vi "getData.vi"(10 "TVAC Labview":bool, 11 "Local Debug":bool) -> ()   [LabVIEW 2017]
uses:
  <vilib>/httpClient/ClientHandle.ctl
  msg7171_linux.llb/send single message.vi
  msg7171_linux.llb/send multiple messages.vi
  <vilib>/httpClient/LabVIEWHTTPClient.lvlib
panel:
  in  "exit":bool
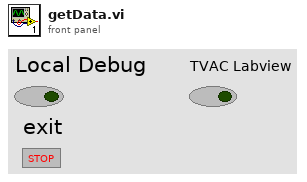
[diagram p1: front panel]
types:
  T1 = typedef "LabVIEWHTTPClient.lvlib/ClientHandle.ctl" = refnum<k1>
  T2 = cluster{"go":bool, "Http session":T1, "URL prefex":string}
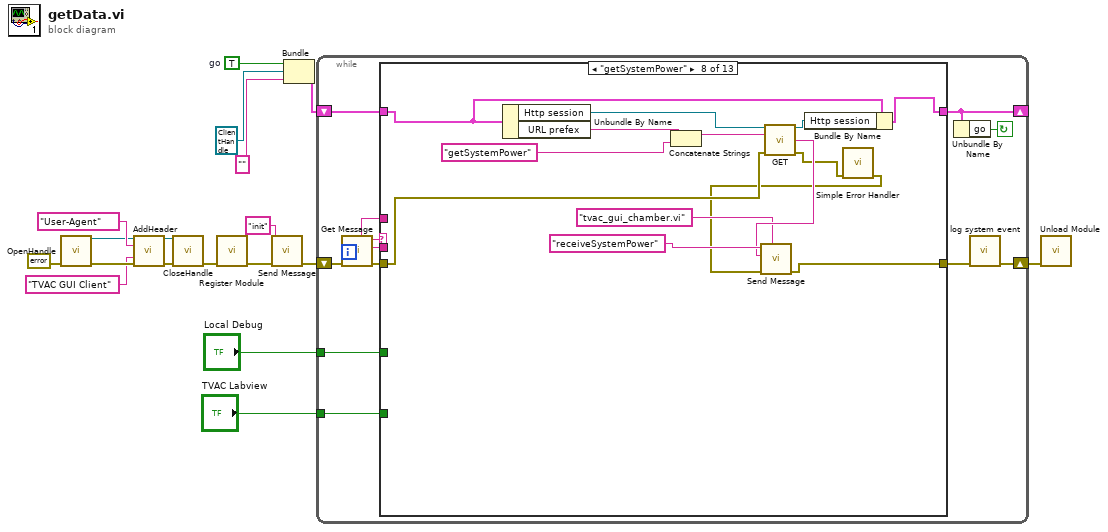
[diagram p0: block diagram]
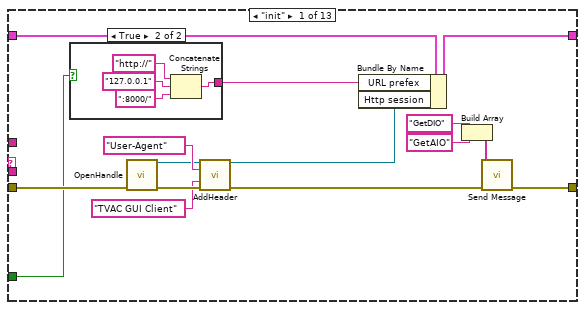
[diagram p2: hidden frame]
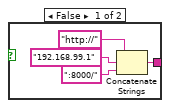
[diagram p3: hidden frame]
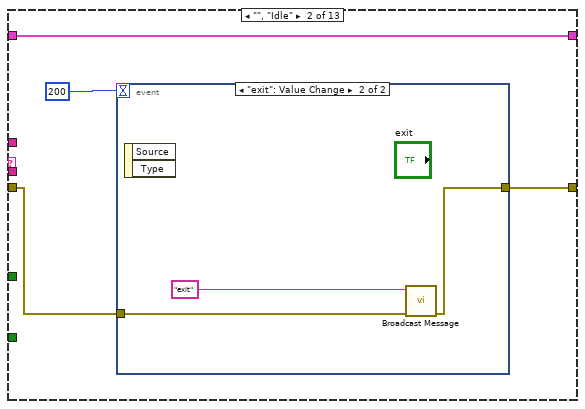
[diagram p4: hidden frame]
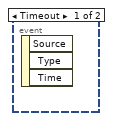
[diagram p5: hidden frame]
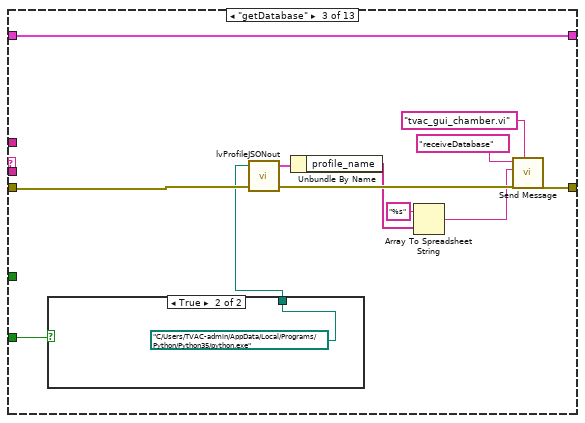
[diagram p6: hidden frame]
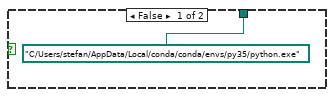
[diagram p7: hidden frame]
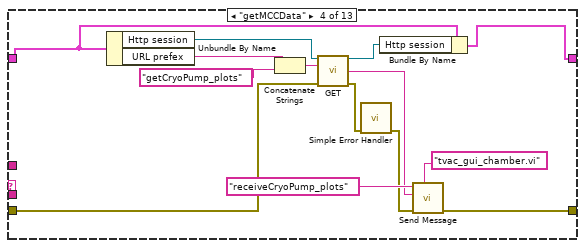
[diagram p8: hidden frame]
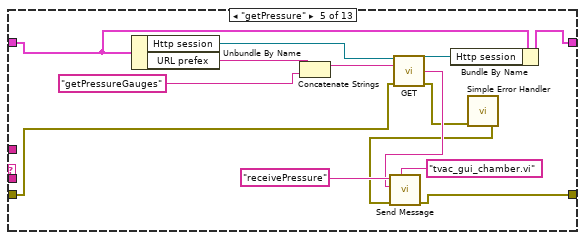
[diagram p9: hidden frame]
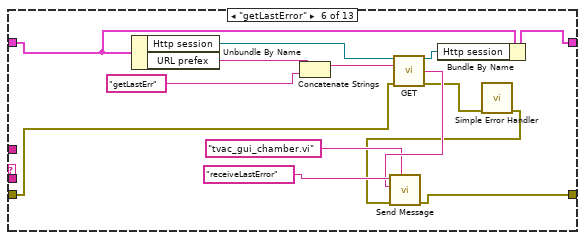
[diagram p10: hidden frame]
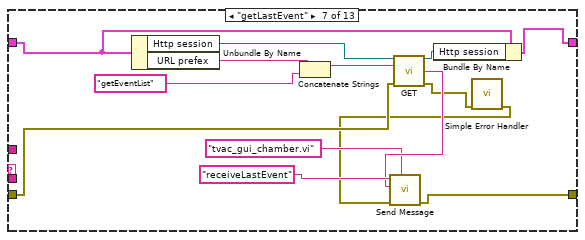
[diagram p11: hidden frame]
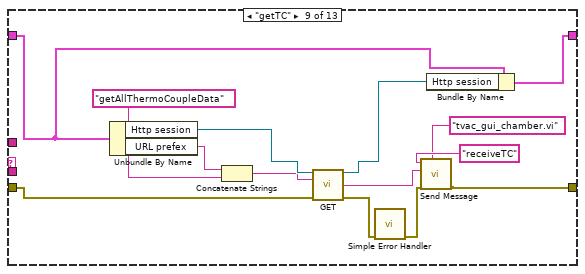
[diagram p12: hidden frame]
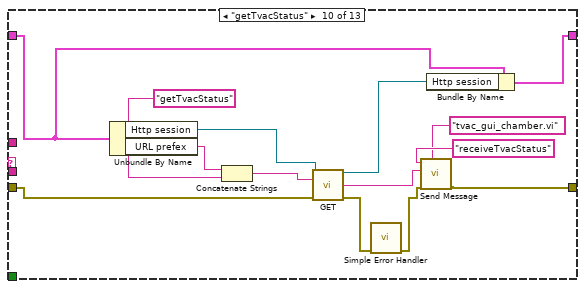
[diagram p13: hidden frame]
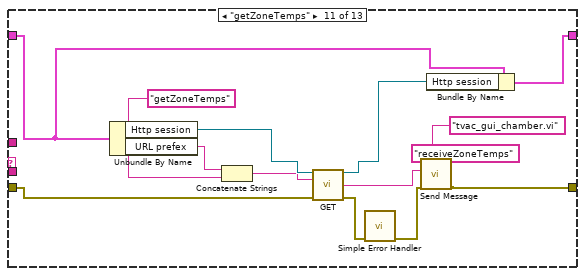
[diagram p14: hidden frame]
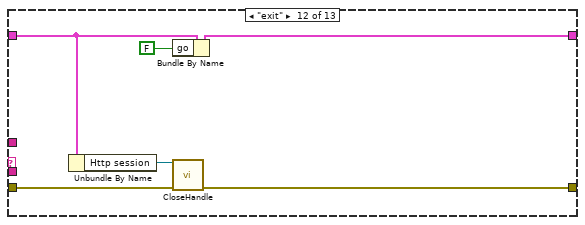
[diagram p15: hidden frame]
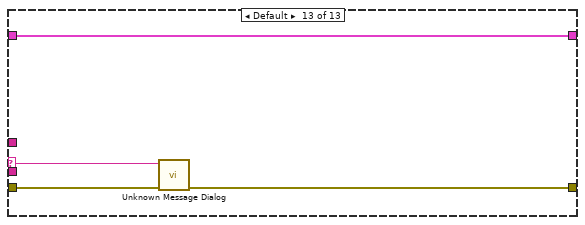
[diagram p16: hidden frame]
diagram:
  w16 = TRUE  # go
  n1 = call <vilib>:"OpenHandle.vi"("error in (no error)"=errorcluster {"status"=FALSE, "code"=0, "source"=""}) -> ("client handle out"=w5:T1, "error out"=w8:errorcluster)  [unwired: 13 in]
  n2 = call <vilib>:"AddHeader.vi"("client handle"=w5, "header"="User-Agent", "value"="TVAC GUI Client", "error in (no error)"=w8) -> ("client handle out"=w4:T1, "error out"=w2:errorcluster)  [unwired: 10 in]
  n3 = call <vilib>:"CloseHandle.vi"("client handle"=w4, "error in (no error)"=w2) -> ("error out"=w3:errorcluster)  [unwired: 13 in]
  n4 = call "Register Module.vi"("error in (no error)"=w3) -> ("error out"=w12:errorcluster)  [unwired: 9 in, 1 out]
  n5 = call-poly "Send Message.vi"("error in (no error)"=w12, "event"="init") -> ("error out"=w11:errorcluster)  [unwired: 9 in]
  n6 = Bundle("go"=w16, "Http session"=T1 refnum, "URL prefex"="") -> (w18:T2)  [unwired: 1 in]
  n7 = while {
    shift-left: w18 -> [w27]
    shift-right: [w25] -> _
    shift-right: [w23] -> w17
    shift-left: w11 -> [w30]
    tunnel: "Local Debug" -> [w20]
    tunnel: "TVAC Labview" -> [w19]
    stop <- w24 continue-if-true
    n8 = call "Get Message.vi"("error in (no error)"=w30) -> ("error out"=w28:errorcluster, "event buffer"=w29:string, "event"=w26:string, "source"=w21:string)  [unwired: 7 in]
    n9 = case shown="\"getSystemPower\"" w26 {
      selector: w26 -> [_ _ _ _ _ _ _ _ _ _ _ _ w194]
      tunnel: [w39 w55 w72 w79 w91 w105 w119 w133 w152 w166 w180 w192 w196] -> w25
      tunnel: w27 -> [w45 w55 w72 w80 w92 w107 w120 w134 w154 w168 w182 w187 w196]
      tunnel: w29 -> [_ _ _ _ _ _ _ _ _ _ _ _ _]
      tunnel: w28 -> [w40 w57 w71 w77 w98 w112 w126 w140 w155 w169 w183 w190 w195]
      tunnel: [w35 w56 w69 w85 w97 w111 w125 w139 w151 w165 w179 w189 w193] -> w22
      tunnel: w21 -> [_ _ _ _ _ _ _ _ _ _ _ _ _]
      tunnel: w20 -> [w31 _ _ _ _ _ _ _ _ _ _ _ _]
      tunnel: w19 -> [_ _ w66 _ _ _ _ _ _ _ _ _ _]
      frame "init" {
        n10 = case shown="True" w31 {
          tunnel: [w46 w51] -> w38
          frame False {
            n11 = Concatenate Strings("http://" ("url"), "192.168.99.1" ("Address"), ":8000/" ("url")) -> (w46:string)
          }
          frame True {
            n12 = Concatenate Strings("http://" ("url"), "127.0.0.1" ("Address"), ":8000/" ("url")) -> (w51:string)
          }
        }
        n13 = call <vilib>:"OpenHandle.vi"("error in (no error)"=w40) -> ("client handle out"=w41:T1, "error out"=w44:errorcluster)  [unwired: 13 in]
        n14 = call <vilib>:"AddHeader.vi"("client handle"=w41, "header"="User-Agent", "value"="TVAC GUI Client", "error in (no error)"=w44) -> ("client handle out"=w37:T1, "error out"=w36:errorcluster)  [unwired: 10 in]
        n15 = Bundle By Name(cluster=w45, "URL prefex"=w38, "Http session"=w37) -> (w39:T2)
        n16 = Build Array("GetDIO" ("event"), "GetAIO" ("event")) -> (w33:string[])
        n17 = call-poly "Send Message.vi"("error in (no error)"=w36, "event"=w33) -> ("error out"=w35:errorcluster)  [unwired: 9 in]
      }
      frame "", "Idle" {
        n18 = event shown="[1] \"exit\": Value Change" {
          selector: _ -> [_ _]
          dyn-events: _ -> [_ _]
          timeout: 200 ("Numeric") -> [_ _]
          tunnel: w57 -> [_ w59]
          tunnel: [_ w58] -> w56
          event Timeout {
            n19 = event-data() -> ()  [unwired: 1 in, 3 out]
          }
          event "exit": Value Change {
            n20 = event-data() -> ()  [unwired: 1 in, 2 out]
            n21 = call "Broadcast Message.vi"("error in (no error)"=w59, "event"="exit") -> ("error out"=w58:errorcluster)  [unwired: 9 in]
          }
        }
      }
      frame "getDatabase" {
        n22 = case shown="True" w66 {
          tunnel: [path "C:/Users/stefan/AppData/Local/conda/conda/envs/py35/python.exe" ("Path to Python.exe") path "C:/Users/TVAC-admin/AppData/Local/Programs/Python/Python35/python.exe" ("Path to Python.exe")] -> w65
          frame False {
          }
          frame True {
          }
        }
        n23 = call "lvProfileJSONout.vi"("error in (no error)"=w71, "Path to Python.exe"=w65) -> ("error out"=w70:errorcluster, "Database Profiles"=w64:cluster{"profile_name":string[]})  [unwired: 1 in, 1 out]
        n24 = Unbundle By Name(w64) -> ("profile_name"=w63:string[])
        n25 = Array To Spreadsheet String(array=w63, 3:"%s" ("format string")) -> (spreadsheet string=w62:string)  [unwired: 1 in]
        n26 = call-poly "Send Message.vi"("Destination Module"="tvac_gui_chamber.vi", "error in (no error)"=w70, "event buffer"=w62, "event"="receiveDatabase") -> ("error out"=w69:errorcluster)  [unwired: 7 in]
      }
      frame "getMCCData" {
        n27 = Unbundle By Name(w80) -> ("Http session"=w81:T1, "URL prefex"=w83:string)
        n28 = Concatenate Strings(w83, "getCryoPump_plots" ("url")) -> (w84:string)
        n29 = call <vilib>:"GET.vi"("client handle"=w81, "url"=w84, "error in (no error)"=w77) -> ("client handle out"=w78:T1, "body"=w87:string, "error out"=w76:errorcluster)  [unwired: 9 in, 1 out]
        n30 = call <vilib>:"Simple Error Handler.vi"("error in (no error)"=w76) -> ("error out"=w75:errorcluster)  [unwired: 4 in, 4 out]
        n31 = Bundle By Name(cluster=w80, "Http session"=w78) -> (w79:T2)
        n32 = call-poly "Send Message.vi"("Destination Module"="tvac_gui_chamber.vi", "error in (no error)"=w75, "event buffer"=w87, "event"="receiveCryoPump_plots" ("url")) -> ("error out"=w85:errorcluster)  [unwired: 7 in]
      }
      frame "getPressure" {
        n33 = Unbundle By Name(w92) -> ("Http session"=w99:T1, "URL prefex"=w101:string)
        n34 = Concatenate Strings(w101, "getPressureGauges" ("url")) -> (w102:string)
        n35 = call <vilib>:"GET.vi"("client handle"=w99, "url"=w102, "error in (no error)"=w98) -> ("client handle out"=w93:T1, "body"=w95:string, "error out"=w90:errorcluster)  [unwired: 9 in, 1 out]
        n36 = Bundle By Name(cluster=w92, "Http session"=w93) -> (w91:T2)
        n37 = call <vilib>:"Simple Error Handler.vi"("error in (no error)"=w90) -> ("error out"=w89:errorcluster)  [unwired: 4 in, 4 out]
        n38 = call-poly "Send Message.vi"("Destination Module"="tvac_gui_chamber.vi", "error in (no error)"=w89, "event buffer"=w95, "event"="receivePressure" ("url")) -> ("error out"=w97:errorcluster)  [unwired: 7 in]
      }
      frame "getLastError" {
        n39 = Unbundle By Name(w107) -> ("Http session"=w113:T1, "URL prefex"=w115:string)
        n40 = Concatenate Strings(w115, "getLastErr" ("url")) -> (w116:string)
        n41 = call <vilib>:"GET.vi"("client handle"=w113, "url"=w116, "error in (no error)"=w112) -> ("client handle out"=w106:T1, "body"=w109:string, "error out"=w104:errorcluster)  [unwired: 9 in, 1 out]
        n42 = Bundle By Name(cluster=w107, "Http session"=w106) -> (w105:T2)
        n43 = call <vilib>:"Simple Error Handler.vi"("error in (no error)"=w104) -> ("error out"=w103:errorcluster)  [unwired: 4 in, 4 out]
        n44 = call-poly "Send Message.vi"("Destination Module"="tvac_gui_chamber.vi", "error in (no error)"=w103, "event buffer"=w109, "event"="receiveLastError" ("url")) -> ("error out"=w111:errorcluster)  [unwired: 7 in]
      }
      frame "getLastEvent" {
        n45 = Unbundle By Name(w120) -> ("Http session"=w127:T1, "URL prefex"=w129:string)
        n46 = Concatenate Strings(w129, "getEventList" ("url")) -> (w130:string)
        n47 = call <vilib>:"GET.vi"("client handle"=w127, "url"=w130, "error in (no error)"=w126) -> ("client handle out"=w121:T1, "body"=w123:string, "error out"=w118:errorcluster)  [unwired: 9 in, 1 out]
        n48 = Bundle By Name(cluster=w120, "Http session"=w121) -> (w119:T2)
        n49 = call <vilib>:"Simple Error Handler.vi"("error in (no error)"=w118) -> ("error out"=w117:errorcluster)  [unwired: 4 in, 4 out]
        n50 = call-poly "Send Message.vi"("Destination Module"="tvac_gui_chamber.vi", "error in (no error)"=w117, "event buffer"=w123, "event"="receiveLastEvent" ("url")) -> ("error out"=w125:errorcluster)  [unwired: 7 in]
      }
      frame "getSystemPower" {
        n51 = Unbundle By Name(w134) -> ("Http session"=w141:T1, "URL prefex"=w143:string)
        n52 = Concatenate Strings(w143, "getSystemPower" ("url")) -> (w144:string)
        n53 = call <vilib>:"GET.vi"("client handle"=w141, "url"=w144, "error in (no error)"=w140) -> ("client handle out"=w135:T1, "body"=w137:string, "error out"=w132:errorcluster)  [unwired: 9 in, 1 out]
        n54 = Bundle By Name(cluster=w134, "Http session"=w135) -> (w133:T2)
        n55 = call <vilib>:"Simple Error Handler.vi"("error in (no error)"=w132) -> ("error out"=w131:errorcluster)  [unwired: 4 in, 4 out]
        n56 = call-poly "Send Message.vi"("Destination Module"="tvac_gui_chamber.vi", "error in (no error)"=w131, "event buffer"=w137, "event"="receiveSystemPower" ("url")) -> ("error out"=w139:errorcluster)  [unwired: 7 in]
      }
      frame "getTC" {
        n57 = Unbundle By Name(w154) -> ("Http session"=w158:T1, "URL prefex"=w147:string)
        n58 = Concatenate Strings(w147, "getAllThermoCoupleData" ("url")) -> (w157:string)
        n59 = call <vilib>:"GET.vi"("client handle"=w158, "url"=w157, "error in (no error)"=w155) -> ("client handle out"=w153:T1, "body"=w149:string, "error out"=w146:errorcluster)  [unwired: 9 in, 1 out]
        n60 = call <vilib>:"Simple Error Handler.vi"("error in (no error)"=w146) -> ("error out"=w145:errorcluster)  [unwired: 4 in, 4 out]
        n61 = call-poly "Send Message.vi"("Destination Module"="tvac_gui_chamber.vi", "error in (no error)"=w145, "event buffer"=w149, "event"="receiveTC" ("url")) -> ("error out"=w151:errorcluster)  [unwired: 7 in]
        n62 = Bundle By Name(cluster=w154, "Http session"=w153) -> (w152:T2)
      }
      frame "getTvacStatus" {
        n63 = Unbundle By Name(w168) -> ("Http session"=w172:T1, "URL prefex"=w161:string)
        n64 = Concatenate Strings(w161, "getTvacStatus" ("url")) -> (w171:string)
        n65 = call <vilib>:"GET.vi"("client handle"=w172, "url"=w171, "error in (no error)"=w169) -> ("client handle out"=w167:T1, "body"=w163:string, "error out"=w160:errorcluster)  [unwired: 9 in, 1 out]
        n66 = call <vilib>:"Simple Error Handler.vi"("error in (no error)"=w160) -> ("error out"=w159:errorcluster)  [unwired: 4 in, 4 out]
        n67 = call-poly "Send Message.vi"("Destination Module"="tvac_gui_chamber.vi", "error in (no error)"=w159, "event buffer"=w163, "event"="receiveTvacStatus" ("url")) -> ("error out"=w165:errorcluster)  [unwired: 7 in]
        n68 = Bundle By Name(cluster=w168, "Http session"=w167) -> (w166:T2)
      }
      frame "getZoneTemps" {
        n69 = Unbundle By Name(w182) -> ("Http session"=w186:T1, "URL prefex"=w175:string)
        n70 = Concatenate Strings(w175, "getZoneTemps" ("url")) -> (w185:string)
        n71 = call <vilib>:"GET.vi"("client handle"=w186, "url"=w185, "error in (no error)"=w183) -> ("client handle out"=w181:T1, "body"=w177:string, "error out"=w174:errorcluster)  [unwired: 9 in, 1 out]
        n72 = call <vilib>:"Simple Error Handler.vi"("error in (no error)"=w174) -> ("error out"=w173:errorcluster)  [unwired: 4 in, 4 out]
        n73 = call-poly "Send Message.vi"("Destination Module"="tvac_gui_chamber.vi", "error in (no error)"=w173, "event buffer"=w177, "event"="receiveZoneTemps" ("url")) -> ("error out"=w179:errorcluster)  [unwired: 7 in]
        n74 = Bundle By Name(cluster=w182, "Http session"=w181) -> (w180:T2)
      }
      frame "exit" {
        n75 = Unbundle By Name(w187) -> ("Http session"=w188:T1)
        n76 = Bundle By Name(cluster=w187, "go"=FALSE ("Bundle Element")) -> (w192:T2)
        n77 = call <vilib>:"CloseHandle.vi"("client handle"=w188, "error in (no error)"=w190) -> ("error out"=w189:errorcluster)  [unwired: 13 in]
      }
      frame Default {
        n78 = call "Unknown Message Dialog.vi"("error in (no error)"=w195, "event name"=w194) -> ("error out"=w193:errorcluster)  [unwired: 9 in]
      }
    }
    n79 = Unbundle By Name(w25) -> ("go"=w24:bool)
    n80 = call "log system event.vi"("error in (no error)"=w22) -> ("error out"=w23:errorcluster)  [unwired: 9 in, 1 out]
  }
  n81 = call "Unload Module.vi"("error in (no error)"=w17) -> ()  [unwired: 10 in, 1 out]
